vi "Create Frame Pattern Script.vi"(8 "error in (no error)":errorcluster, 9 "ChipID":u8, 10 "Frame_Data":T1={"Pattern_Name"="", "Operation Mode"=enum."Normal", "BurstLength"=enum."0", "FSN"=0, "Start_Addr"=0, "Data"=[], "R/W?"=enum."Read", "Opcode"=[], "ChipID"=1, "num of wait cycle of read"=0} {"Data" format="%x"; "Start_Addr" format="%x"}, 11 "BML_Frame_RW in":refnum<class "BML_Frame_RW.lvclass">) -> (0 "error out":errorcluster, 3 "BML_Frame_RW out":refnum<class "BML_Frame_RW.lvclass">)   [LabVIEW 2018, in "BML_Frame_RW.lvclass"]
uses:
  BML_Frame_RW.lvclass
  C:/P4 Workspace/PC Client/Solutions/5g_eap/HiSi/trunk/1.0/BML_Pattern_Gen_Refactor/Classes/BML_Frame_Root/BML_Frame_Root.lvclass
  Config_Read/Frame_Data.ctl
  Config_Read/OperationMode.ctl
  Config_Read/BurstLength.ctl
  Config_Read/RW_Option.ctl
  BML_Frame_Root/Special Frame.ctl
  BML_Frame_RW.lvclass/BML_Frame_RW.ctl
  BML_Frame_Root/BML_Frame_Root.lvclass/BML_Frame_Root.ctl
  BML_Frame_Write/BML_Frame_Write.lvclass
  BML_Frame_ReadData_Compare/BML_Frame_ReadData_Compare.lvclass
  BML_Frame_ReadCollect/BML_Frame_ReadCollect.lvclass
  BML_Frame_Root/BML_Frame_Root.lvclass
  Config_Read/Config_Read_BML.lvclass
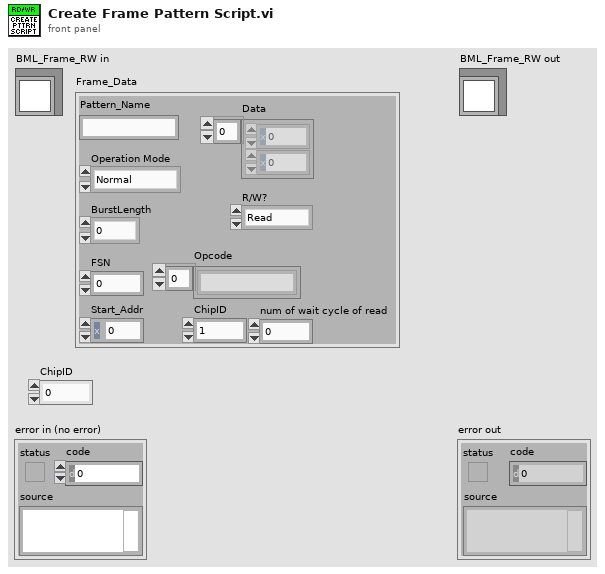
[diagram p1: front panel]
types:
  T1 = typedef "Config_Read_BML.lvclass/Frame_Data.ctl" = cluster{"Pattern_Name":string, "Operation Mode":T2, "BurstLength":T3, "FSN":u8, "Start_Addr":u16, "Data":u8[], "R/W?":T4, "Opcode":string[], "ChipID":u8, "num of wait cycle of read":i8}
  T2 = typedef "Config_Read_BML.lvclass/OperationMode.ctl" = enum8{"Normal", "ImmeEffect", "InitSlaveID", "LoadData"}
  T3 = typedef "Config_Read_BML.lvclass/BurstLength.ctl" = enum8{"0", "2", "3", "4", "5", "8", "16", "32"}
  T4 = typedef "Config_Read_BML.lvclass/RW_Option.ctl" = enum16{"Read", "Write", "R/W"}
  T5 = typedef "BML_Frame_Root.lvclass/Special Frame.ctl" = enum16{"Sync Header", "Protocol Header", "SW Trig", "SetID State", "Out SetID State", "SW Reset", "Wait", "SPI 4W FRM Start", "SPI 4W Wait", "SPI 4W FRM End", "SPI 4W Write Cmd", "SPI RD Collect Cmd", "SPI RD Value Cmd", "SPI 3W FRM Start", "SPI 3W Write Cmd", "SPI 3W FRM End", "SPI 3W Wait", "SPI 3W RD Cmd"}
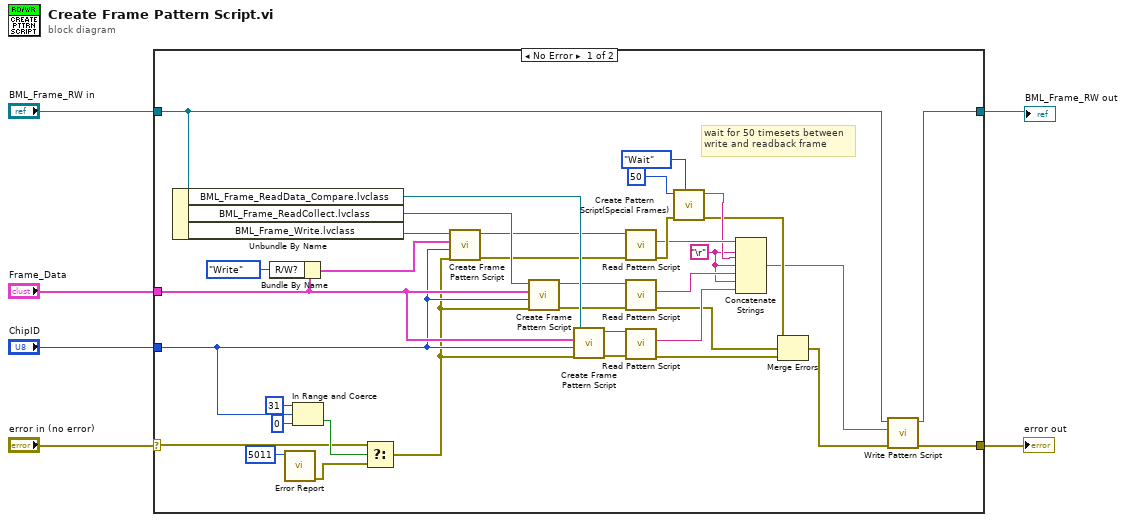
[diagram p0: block diagram]
diagram:
  n1 = case shown="No Error" "error in (no error)" {
    selector: "error in (no error)" -> [w10 w44]
    tunnel: [w19 w44] -> w5
    tunnel: "BML_Frame_RW in" -> [w20 w43]
    tunnel: [w18 w43] -> w3
    tunnel: "Frame_Data" -> [w17 _]
    tunnel: "ChipID" -> [w9 _]
    frame No Error {
      w27 = "\r"
      # "wait for 50 timesets between\nwrite and readback frame"
      n2 = Unbundle By Name(w20) -> ("BML_Frame_ReadData_Compare.lvclass"=w40:refnum<class "BML_Frame_ReadData_Compare.lvclass">, "BML_Frame_ReadCollect.lvclass"=w41:refnum<class "BML_Frame_ReadCollect.lvclass">, "BML_Frame_Write.lvclass"=w42:refnum<class "BML_Frame_Write.lvclass">)
      n3 = Bundle By Name(cluster=w17, "R/W?"=RW_Option."Write") -> (w15:T1)
      n4 = call "Error Report.vi"("Error Code"=i16 5011) -> ("error out"=w8:errorcluster)  [unwired: 10 in]
      n5 = In Range and Coerce(upper limit=u8 31, x=w9, lower limit=u8 0) -> (In Range?=w12:bool)  [unwired: 1 out]
      n6 = Select(t=w10, s=w12, f=w8) -> (s? t:f=w7:errorcluster)
      n7 = call-dynamic "Create Frame Pattern Script.vi"("error in (no error)"=w7, "ChipID"=w9, "Frame_Data"=w15, "BML_Frame_Write in"=w42) -> ("error out"=w39:errorcluster, "BML_Frame_Write out"=w38:refnum<class "BML_Frame_Write.lvclass">)  [unwired: 6 in]
      n8 = call-dynamic "Create Frame Pattern Script.vi"("error in (no error)"=w7, "ChipID"=w9, "Frame_Data"=w17, "BML_Frame_ReadCollect in"=w41) -> ("error out"=w36:errorcluster, "BML_Frame_ReadCollect out"=w37:refnum<class "BML_Frame_ReadCollect.lvclass">)  [unwired: 6 in]
      n9 = call-dynamic "Create Frame Pattern Script.vi"("error in (no error)"=w7, "ChipID"=w9, "Frame_Data"=w17, "BML_Frame_ReadData_Compare in"=w40) -> ("error out"=w35:errorcluster, "BML_Frame_ReadData_Compare out"=w34:refnum<class "BML_Frame_ReadData_Compare.lvclass">)  [unwired: 6 in]
      n10 = call "Read Pattern Script.vi"("error in (no error)"=w39, "BML_Frame_Root in"=w38) -> ("error out"=w33:errorcluster, "Pattern Script"=w30:string)  [unwired: 7 in, 1 out]
      n11 = call "Read Pattern Script.vi"("error in (no error)"=w36, "BML_Frame_Root in"=w37) -> ("error out"=w24:errorcluster, "Pattern Script"=w28:string)  [unwired: 7 in, 1 out]
      n12 = call "Read Pattern Script.vi"("error in (no error)"=w35, "BML_Frame_Root in"=w34) -> ("error out"=w23:errorcluster, "Pattern Script"=w26:string)  [unwired: 7 in, 1 out]
      n13 = call "Create Pattern Script(Special Frames).vi"("Special Frame Type"=Special_Frame."Wait", "error in (no error)"=w33, "Num of Timeset"=u32 50) -> ("error out"=w25:errorcluster, "string out"=w29:string)  [unwired: 7 in]
      n14 = Concatenate Strings(w30, w27, w29, w27, w28, w27, w26) -> (w21:string)
      n15 = Merge Errors(w25, w24, w23) -> (w22:errorcluster)
      n16 = call "Write Pattern Script.vi"("error in (no error)"=w22, "Pattern Script"=w21, "BML_Frame_Root in"=w20) -> ("error out"=w19:errorcluster, "BML_Frame_Root out"=w18:refnum<class "BML_Frame_RW.lvclass">)  [unwired: 7 in]
    }
    frame Error {
    }
  }
  "error out" <- w5
  "BML_Frame_RW out" <- w3
